vi "Conditional Map of U32 to U32.vi"(1 "map in":map{u32, u32}(c390)) -> (0 "Boolean":bool)   [LabVIEW 2020]
doc: "Monitors a map. The Data tab displays the size of the map and its contents. Use the Conditions tab to set a conditional breakpoint. You can set conditions based on the size of the map and/or its contents. If you select multiple conditions, LabVIEW executes a breakpoint if any of those conditions are true."
uses:
  0355159d-d0e7-4984-8129-25129ee27db6.vi
panel:
  in  "Tab Control":enum32{"Data   ", "Conditions      "}(tab)
  out "Map":map{u32, u32}(c390)
  in  "Does not contain a key":bool
  in  "Contains a key":bool
  in  "Number of Elements Condition":u16(ring) items=["Equal to", "Greater than", "Less than"]
  in  "Number of elements value":u32
  in  "Number of elements is":bool
  in  "Contains":u32
  in  "Does Not Contain":u32
  # "Pause if any of the following:"
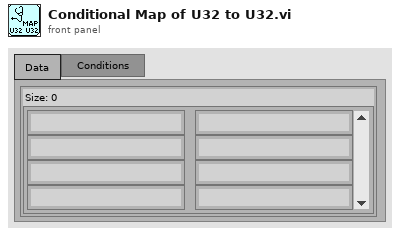
[diagram p1: front panel]
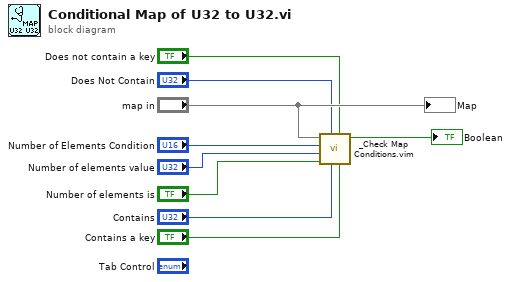
[diagram p0: block diagram]
diagram:
  n1 = call "_Check Map Conditions.vim"("Contains key"="Contains a key", "Does not contain key"="Does not contain a key", "contains"="Contains", "does not contain"="Does Not Contain", "# elements"="Number of elements is", "# elements value"="Number of elements value", "# elements condition"="Number of Elements Condition", "map"="map in") -> ("Pause"=→"Boolean":bool)  [unwired: 3 in]
  "Map" <- "map in"
